vi "StartingLocations.vi"(11 "Index":i32) -> (3 "Location":cluster{dbl, dbl})   [LabVIEW 2018]
uses:
  Robot-Project/Configuration/Constants.vi
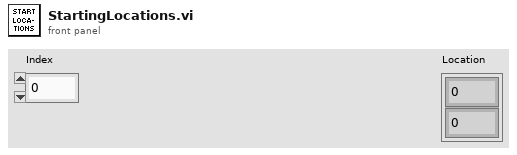
[diagram p1: front panel]
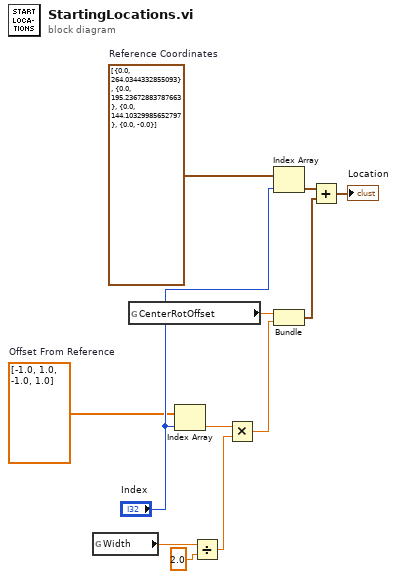
[diagram p0: block diagram]
diagram:
  w6 = dbl[] [-1.0, 1.0, -1.0, 1.0]  # Offset From Reference
  w7 = cluster{dbl, dbl}[] [{0.0, 264.0344332855093}, {0.0, 195.23672883787663}, {0.0, 144.10329985652797}, {0.0, -0.0}]  # Reference Coordinates
  n1 = global read "Constants.vi" "Width"() -> (w4:dbl)
  n2 = global read "Constants.vi" "CenterRotOffset"() -> (w2:dbl)
  n3 = Index Array(array=w6, index="Index") -> (element=w10:dbl)
  n4 = Divide(x=w4, y=2.0) -> (x/y=w5:dbl)
  n5 = Multiply(x=w10, y=w5) -> (x*y=w11:dbl)
  n6 = Index Array(array=w7, index="Index") -> (element=w8:cluster{dbl, dbl})
  n7 = Bundle("CenterRotOffset"=w2, w11) -> (w12:cluster{"CenterRotOffset":dbl, dbl})  [unwired: 1 in]
  n8 = Add(x=w8, y=w12) -> (x+y=→"Location":cluster{dbl, dbl})
